vi "Com_SECS Equipment _Stream_S1F3.vi"(8 "error in":errorcluster, 11 "Status Variable ID(SVID)":u32[](array[numeric])) -> (0 "error out":errorcluster, 3 "SECS Packet":T1)   [LabVIEW 2016]
uses:
  Data Def/Com_SECS Equipment _SECS Packet.ctl
  Data Def/Com_SECS Equipment _Message Type.ctl
  Data Def/Com_SECS Equipment _Protocol Type.ctl
  Data Def/Com_SECS Equipment _Stream Type.ctl
  Data Def/Com_SECS Equipment _Build Message Setting.ctl
  Data Message/Com_SECS Equipment _Data Message_List.vi
  Data Message/Com_SECS Equipment _Data Message_U4.vi
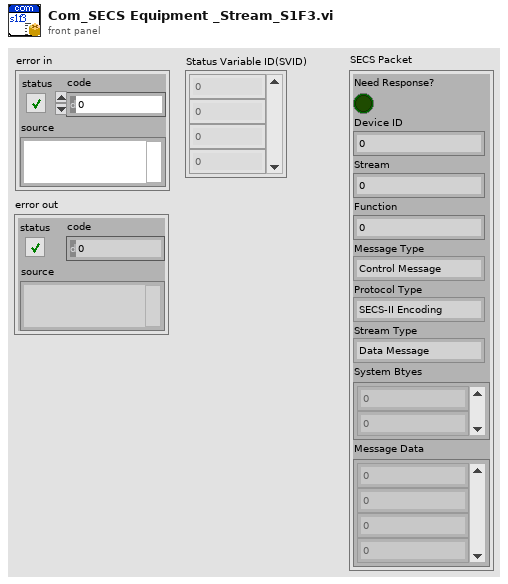
[diagram p1: front panel]
types:
  T1 = typedef "Com_SECS Equipment _SECS Packet.ctl" = cluster{"Need Response?":bool, "Device ID":u16, "Stream":u8, "Function":u8, "Message Type":T2, "Protocol Type":T3, "Stream Type":T4, "System Btyes":u8[], "Message Data":u8[]}
  T2 = typedef "Com_SECS Equipment _Message Type.ctl" = enum16{"Control Message", "Data Message"}
  T3 = typedef "Com_SECS Equipment _Protocol Type.ctl" = enum16{"SECS-II Encoding", "Reserved"}
  T4 = typedef "Com_SECS Equipment _Stream Type.ctl" = enum16{"Data Message", "Select.req", "Select.rsp", "Deselect.req", "Deselect.rsp", "Linktest.req", "Linktest.rsp", "Reject.req", "Separate.req", "Reserve"}
  T5 = typedef "Com_SECS Equipment _Build Message Setting.ctl" = cluster{"Stream":u8, "Function":u8, "Need Response?":bool}
  T6 = typedef "Com_SECS Equipment _Message Data.ctl" = cluster{"Index":i32, "Data Item Format":T7, "Format Code":T8, "Parent Index":i32, "Child Index":i32[], "Data":variant}
  T7 = typedef "Com_SECS Equipment _Data Item Format.ctl" = enum16{"Data Type", "Value"}
  T8 = typedef "Com_SECS Equipment _Format Code.ctl" = enum16{"L", "A", "B", "Boolean", "J", "I1", "I2", "I4", "I8", "U1", "U2", "U4", "U8", "F4", "F8", "Char"}
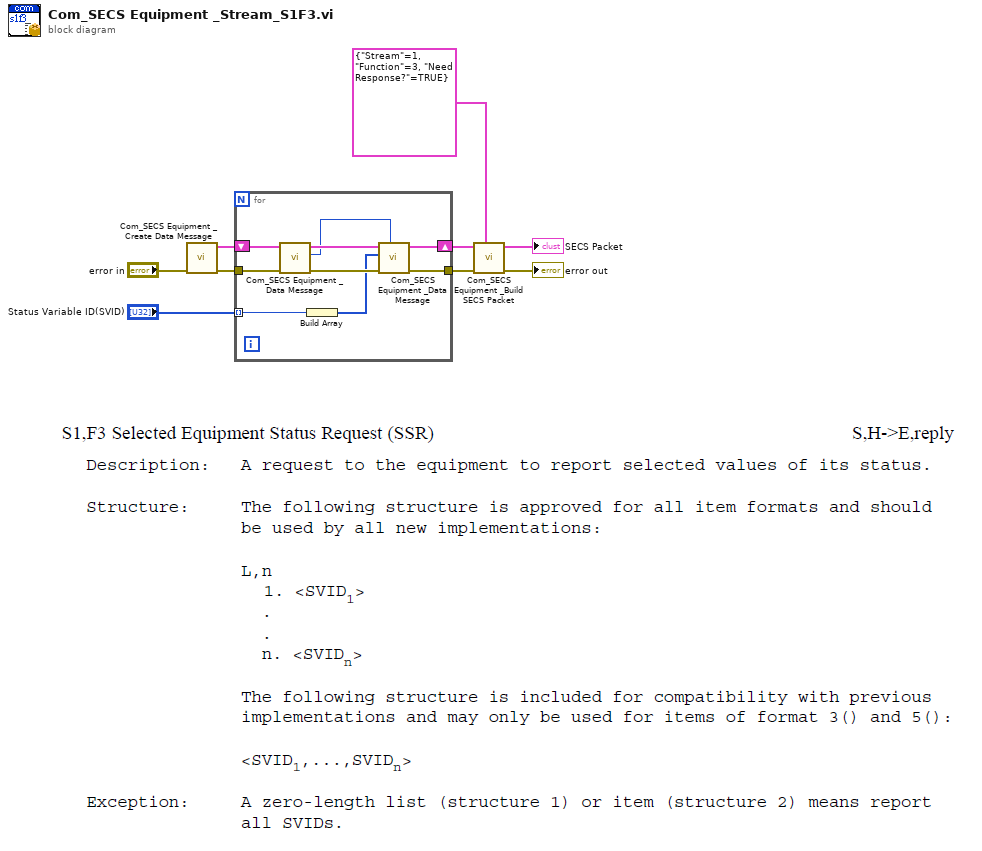
[diagram p0: block diagram]
diagram:
  n1 = call "Com_SECS Equipment _Create Data Message.vi"("error in"="error in") -> ("error out"=w5:errorcluster, "Message Data"=w4:T6[])  [unwired: 9 in]
  n2 = for {
    tunnel: w5 -> [w18]
    tunnel: "Status Variable ID(SVID)" -> [w13] mode=indexing
    shift-right: [w11] -> w2
    shift-left: w4 -> [w17]
    tunnel: [w10] -> w1
    n3 = call-poly "Com_SECS Equipment _Data Message.vi"("error in"=w18, "Message Data In"=w17) -> ("error out"=w16:errorcluster, "Index"=w14:i32, "Message Data Out"=w15:T6[])  [unwired: 7 in]
    n4 = Build Array(w13) -> (w12:u32[])
    n5 = call-poly "Com_SECS Equipment _Data Message.vi"("Parent Index"=w14, "error in"=w16, "Data"=w12, "Message Data In"=w15) -> ("error out"=w10:errorcluster, "Message Data Out"=w11:T6[])  [unwired: 6 in]
  }
  n6 = call "Com_SECS Equipment _Build SECS Packet.vi"("Build Message Setting"=T5 {"Stream"=1, "Function"=3, "Need Response?"=TRUE}, "error in"=w1, "Message Data"=w2) -> ("error out"=→"error out":errorcluster, "SECS Packet"=→"SECS Packet":T1)  [unwired: 7 in]
